vi "CARRY_MOVE.vi"(6 "ARM 2 FEEDBACK":dbl, 7 "RESET":bool, 8 "ARM 1 FEEDBACK":dbl, 9 "ARM 2 INITIAL":dbl, 10 "ARM 1 INITIAL":dbl, 11 "INPUT":bool) -> (0 "ARM 2 SETPOINT OUT":dbl, 2 "RUNNING?":bool, 3 "ARM 1 SETPOINT OUT":dbl)   [LabVIEW 2017]
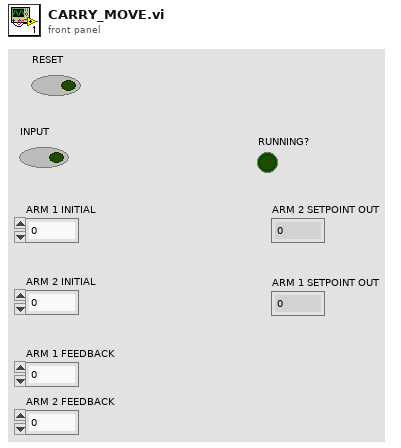
[diagram p1: front panel]
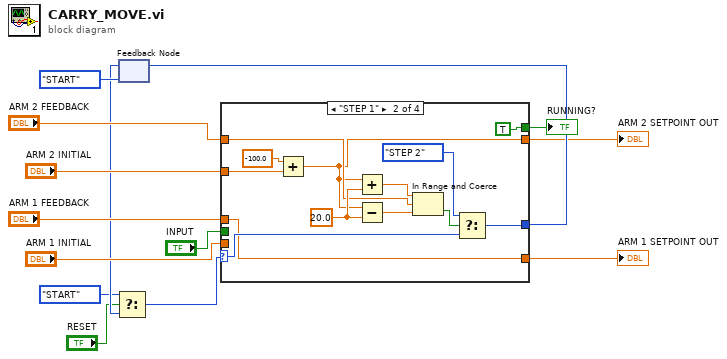
[diagram p0: block diagram]
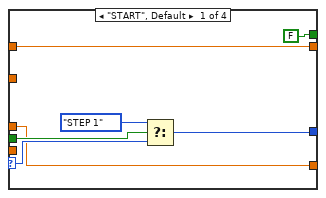
[diagram p2: hidden frame]
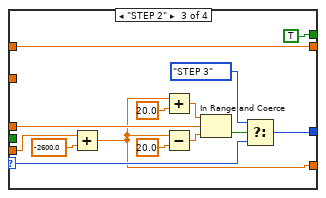
[diagram p3: hidden frame]
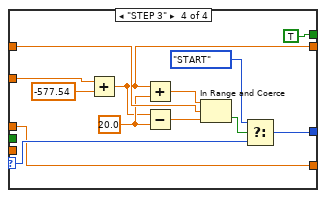
[diagram p4: hidden frame]
diagram:
  n1 = feedback #1(enum16{"START", "STEP 1", "STEP 2", "STEP 3"}."START") -> (w3:enum16{"START", "STEP 1", "STEP 2", "STEP 3"})
  n2 = Select(t=enum16{"START", "STEP 1", "STEP 2", "STEP 3"}."START", s="RESET", f=w3) -> (s? t:f=w4:enum16{"START", "STEP 1", "STEP 2", "STEP 3"})
  n3 = case shown="\"STEP 1\"" w4 {
    selector: w4 -> [w20 w34 w48 w61]
    tunnel: [w21 w33 w47 w60] -> w13
    tunnel: "INPUT" -> [w19 _ _ _]
    tunnel: "ARM 1 INITIAL" -> [_ _ w36 _]
    tunnel: "ARM 2 INITIAL" -> [_ w24 _ w50]
    tunnel: "ARM 2 FEEDBACK" -> [w16 w25 w39 w55]
    tunnel: [w16 w23 w39 w49] -> w8
    tunnel: "ARM 1 FEEDBACK" -> [w17 w26 w38 w58]
    tunnel: [w17 w26 w35 w58] -> w6
    tunnel: [FALSE TRUE TRUE TRUE] -> w5
    frame "START", Default {
      n4 = Select(t=enum16{"START", "STEP 1", "STEP 2", "STEP 3"}."STEP 1", s=w19, f=w20) -> (s? t:f=w21:enum16{"START", "STEP 1", "STEP 2", "STEP 3"})
    }
    frame "STEP 1" {
      w27 = 20.0 ("y")
      n5 = Add(x=-100.0, y=w24) -> (x+y=w23:dbl)
      n6 = Add(x=w23, y=w27) -> (x+y=w28:dbl)
      n7 = Subtract(x=w23, y=w27) -> (x-y=w29:dbl)
      n8 = In Range and Coerce(upper limit=w28, x=w25, lower limit=w29) -> (In Range?=w30:bool)  [unwired: 1 out]
      n9 = Select(t=enum16{"START", "STEP 1", "STEP 2", "STEP 3"}."STEP 2", s=w30, f=w34) -> (s? t:f=w33:enum16{"START", "STEP 1", "STEP 2", "STEP 3"})
    }
    frame "STEP 2" {
      n10 = Add(x=w36, y=-2600.0) -> (x+y=w35:dbl)
      n11 = Add(x=w35, y=20.0) -> (x+y=w43:dbl)
      n12 = Subtract(x=w35, y=20.0) -> (x-y=w42:dbl)
      n13 = In Range and Coerce(upper limit=w43, x=w38, lower limit=w42) -> (In Range?=w44:bool)  [unwired: 1 out]
      n14 = Select(t=enum16{"START", "STEP 1", "STEP 2", "STEP 3"}."STEP 3", s=w44, f=w48) -> (s? t:f=w47:enum16{"START", "STEP 1", "STEP 2", "STEP 3"})
    }
    frame "STEP 3" {
      w52 = 20.0 ("y")
      n15 = Add(x=w50, y=-577.54) -> (x+y=w49:dbl)
      n16 = Add(x=w49, y=w52) -> (x+y=w53:dbl)
      n17 = Subtract(x=w49, y=w52) -> (x-y=w54:dbl)
      n18 = In Range and Coerce(upper limit=w53, x=w55, lower limit=w54) -> (In Range?=w56:bool)  [unwired: 1 out]
      n19 = Select(t=enum16{"START", "STEP 1", "STEP 2", "STEP 3"}."START", s=w56, f=w61) -> (s? t:f=w60:enum16{"START", "STEP 1", "STEP 2", "STEP 3"})
    }
  }
  "ARM 2 SETPOINT OUT" <- w8
  "ARM 1 SETPOINT OUT" <- w6
  "RUNNING?" <- w5
  n20 = feedback-in #1(w13) -> ()
